vi "Destroy to Listener.vi"(8 "Error In":errorcluster, 10 "Channel":refnum<class "Channel.lvclass">, 11 "Listener In":refnum<class "Listener.lvclass">) -> (0 "Error Out":errorcluster, 3 "Listener Out":refnum<class "Listener.lvclass">)   [LabVIEW 2021, in "Field_RnD_Services_LIBSSH2_Toolkit.lvlib" / "Channel.lvclass"]
doc: "Passes through the Listener and destroys this Channel object."
uses:
  Channel.lvclass
  Listener/Listener.lvclass
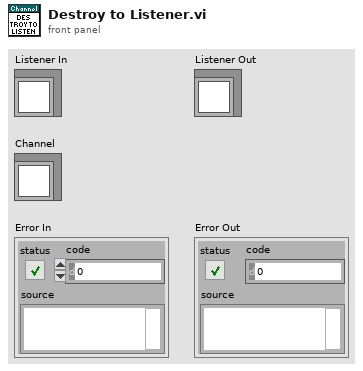
[diagram p1: front panel]
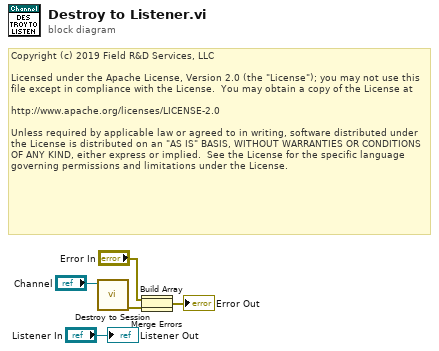
[diagram p0: block diagram]
diagram:
  # "Copyright (c) 2019 Field R&D Services, LLC\n\nLicensed under the Apache License, Version 2.0 (the \"License\"); you may not use this file except in compliance with the License.  You may obtain a copy of the License at\n\nhttp://www.apache.org/licenses/LICENSE-2.0\n\nUnless required by applicable law or agreed to in writing, software distributed under the License is distributed on an \"AS IS\" BASIS, WITHOUT WARRANTIES OR CONDITIONS OF ANY KIND, either express or implied.  See the License for the specific language governing permissions and limitations under the License."
  n1 = call "Destroy to Session.vi"("Channel"="Channel") -> ("Error Out"=w2:errorcluster)  [unwired: 9 in, 1 out]
  n2 = Build Array("Error In", w2) -> (w1:errorcluster[])
  n3 = Merge Errors(w1) -> (→"Error Out":errorcluster)
  "Listener Out" <- "Listener In"
